vi "SACB v0.1.vi"(6 "timeout":i32=50, 7 "Command":enum16{"Create", "Read", "Close"}(ring), 8 "Error In":errorcluster, 11 "Model Name":T1) -> (0 "Error Out":errorcluster, 2 "Connected?":bool, 3 "Digital Inputs":T2)   [LabVIEW 2017]
uses:
  <vilib>/Modbus/master/Modbus Master.lvclass
  <vilib>/Modbus/master/Create Master Instance (TCP).vi
  controls/Model Name.ctl
  controls/SACB DI.ctl
panel:
  out "register values":u16[][](array[numeric])
  # "RS_Clamping_top_Front\nRS_Clamping_bottom_Front\nRS_Clamping_MotorLH_Front\nRS_Clamping_MotorRH_Front\nIPS_Part presence_top_LH\nIPS_Part presence_Bottom_LH\nIPS_Part presence_top_RH\nIPS_Part presence_Bottom_RH\nIPS_Load engaged_1\nIPS_Part presence_2\nIPS_Load engaged_MCO_LH\nIPS_Load engaged_MCO_RH"
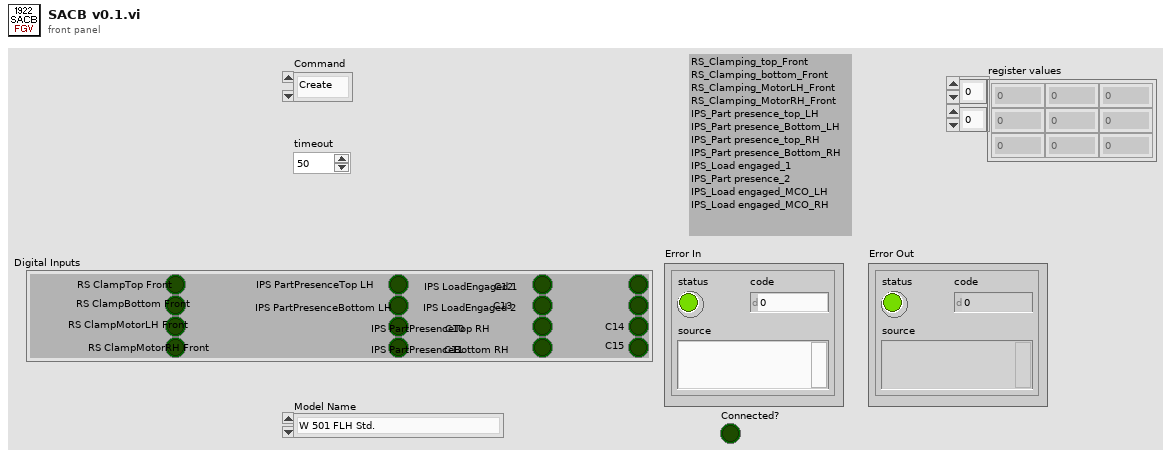
[diagram p1: front panel]
types:
  T1 = typedef "Model Name.ctl" = enum16{"W 501 FLH Std.", "W 501 FRH Std.", "W 601 FR RH Std", "W 601 FR LH Std", "W 601 RR RH Std", "W 601 RR LH Std", "W 601 FR RH AP", "W 601 FR LH AP", "W 601 RR RH AP", "W 601 RR LH AP"}
  T2 = typedef "SACB DI.ctl" = cluster{"RS ClampTop Front":bool, "RS ClampBottom Front":bool, "RS ClampMotorLH Front":bool, "RS ClampMotorRH Front":bool, "IPS PartPresenceTop LH":bool, "IPS PartPresenceBottom LH":bool, "IPS PartPresenceTop RH":bool, "IPS PartPresenceBottom RH":bool, "IPS LoadEngaged 1":bool, "IPS LoadEngaged 2":bool, "C10":bool, "C11":bool, "C12":bool, "C13":bool, "C14":bool, "C15":bool}
  T3 = cluster{"[0]":bool, "[1]":bool, "[2]":bool, "[3]":bool, "[4]":bool, "[5]":bool, "[6]":bool, "[7]":bool, "[8]":bool, "[9]":bool, "[10]":bool, "[11]":bool, "[12]":bool, "[13]":bool, "[14]":bool, "[15]":bool}
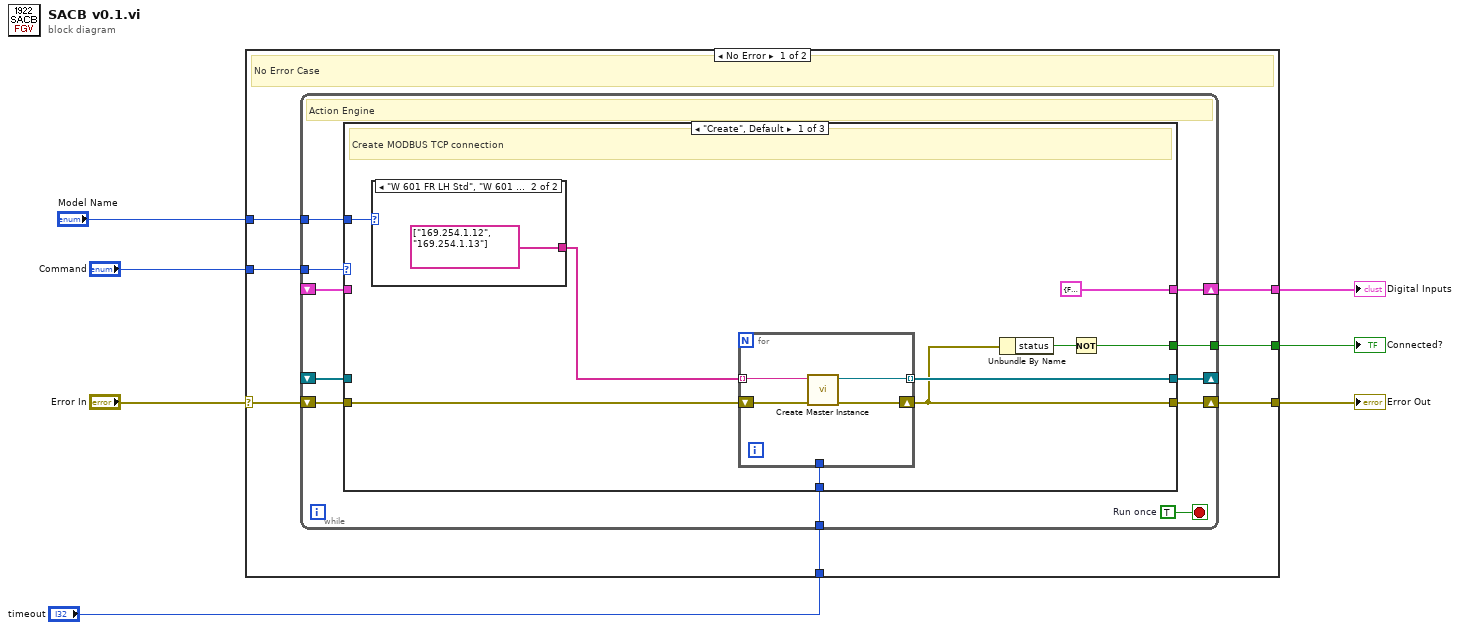
[diagram p0: block diagram]
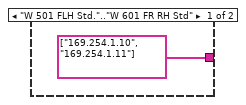
[diagram p2: hidden frame]
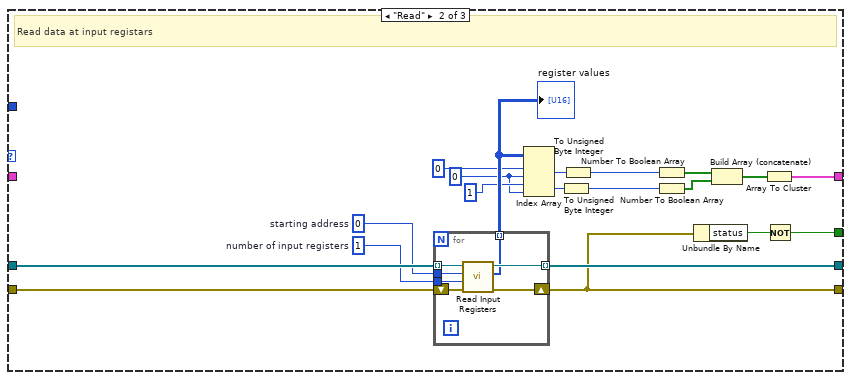
[diagram p3: hidden frame]
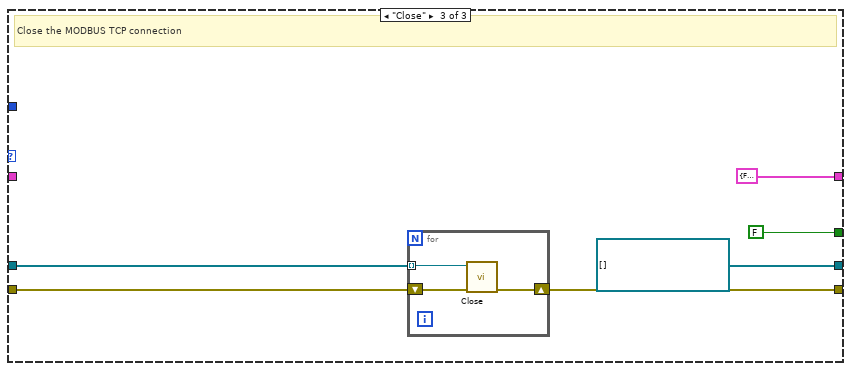
[diagram p4: hidden frame]
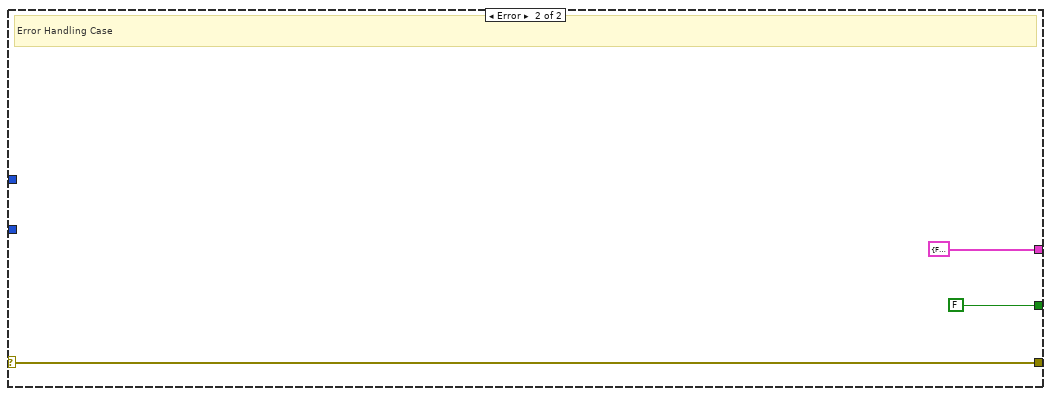
[diagram p5: hidden frame]
diagram:
  n1 = case shown="No Error" "Error In" {
    selector: "Error In" -> [w13 w79]
    tunnel: [w14 w79] -> w6
    tunnel: "Command" -> [w12 _]
    tunnel: [w11 T3 {"[0]"=FALSE, "[1]"=FALSE, "[2]"=FALSE, "[3]"=FALSE, "[4]"=FALSE, "[5]"=FALSE, "[6]"=FALSE, "[7]"=FALSE, "[8]"=FALSE, "[9]"=FALSE, "[10]"=FALSE, "[11]"=FALSE, "[12]"=FALSE, "[13]"=FALSE, "[14]"=FALSE, "[15]"=FALSE}] -> w4
    tunnel: [w10 FALSE] -> w3
    tunnel: "timeout" -> [w9 _]
    tunnel: "Model Name" -> [w8 _]
    frame No Error {
      # "No Error Case"
      n2 = while {
        tunnel: w12 -> [w23]
        shift-right: [w25] -> w14
        shift-left: w13 -> [w24]
        shift-right: [w21] -> _
        shift-left: _ -> [w20]
        shift-right: [w19] -> w11
        shift-left: _ -> [w18]
        tunnel: [w17] -> w10
        tunnel: w9 -> [w16]
        tunnel: w8 -> [w15]
        stop <- w22 stop-if-true
        w22 = TRUE  # Run once
        # "Action Engine"
        n3 = case shown="\"Create\", Default" w23 {
          tunnel: [w31 w46 w72] -> w25
          tunnel: w24 -> [w34 w60 w73]
          tunnel: [w33 w59 refnum<class "Modbus Master.lvclass">[] []] -> w21
          tunnel: w20 -> [_ w58 w71]
          tunnel: [T3 {"[0]"=FALSE, "[1]"=FALSE, "[2]"=FALSE, "[3]"=FALSE, "[4]"=FALSE, "[5]"=FALSE, "[6]"=FALSE, "[7]"=FALSE, "[8]"=FALSE, "[9]"=FALSE, "[10]"=FALSE, "[11]"=FALSE, "[12]"=FALSE, "[13]"=FALSE, "[14]"=FALSE, "[15]"=FALSE} w48 T3 {"[0]"=FALSE, "[1]"=FALSE, "[2]"=FALSE, "[3]"=FALSE, "[4]"=FALSE, "[5]"=FALSE, "[6]"=FALSE, "[7]"=FALSE, "[8]"=FALSE, "[9]"=FALSE, "[10]"=FALSE, "[11]"=FALSE, "[12]"=FALSE, "[13]"=FALSE, "[14]"=FALSE, "[15]"=FALSE}] -> w19
          tunnel: w18 -> [_ _ _]
          tunnel: [w29 w45 FALSE] -> w17
          tunnel: w16 -> [w28 _ _]
          tunnel: w15 -> [w26 _ _]
          frame "Create", Default {
            # "Create MODBUS TCP connection"
            n4 = case shown="\"W 601 FR LH Std\", \"W 601 RR RH Std\"" w26 {
              tunnel: [string[] ["169.254.1.10", "169.254.1.11"] string[] ["169.254.1.12", "169.254.1.13"]] -> w27
              frame "W 501 FLH Std.".."W 601 FR RH Std" {
              }
              frame "W 601 FR LH Std", "W 601 RR RH Std" {
              }
            }
            n5 = for {
              tunnel: [w36] -> w33 mode=indexing
              shift-right: [w38] -> w31
              shift-left: w34 -> [w37]
              tunnel: w27 -> [w35] mode=indexing
              tunnel: w28 -> [_]
              n6 = call-poly <vilib>:"Create Master Instance.vi"("error in (no error)"=w37, "address"=w35) -> ("error out"=w38:errorcluster, "TCP master instance"=w36:refnum<class "Modbus Master.lvclass">)  [unwired: 8 in]
            }
            n7 = Unbundle By Name(w31) -> ("status"=w30:bool)
            n8 = Not(x=w30) -> (.not. x?=w29:bool)
          }
          frame "Read" {
            w43 = 0 ("disabled index (col)")
            w56 = u16 1  # number of input registers
            w57 = u16 0  # starting address
            # "Read data at input registars"
            n9 = for {
              tunnel: [w65] -> w59 mode=indexing
              tunnel: w58 -> [w64] mode=indexing
              tunnel: w57 -> [w63]
              tunnel: w56 -> [w62]
              tunnel: [w61] -> w53 mode=indexing
              shift-right: [w66] -> w46
              shift-left: w60 -> [w67]
              n10 = call-dynamic "Read Input Registers.vi"("error in (no error)"=w67, "number of input registers"=w62, "starting address"=w63, "Modbus master in"=w64) -> ("error out"=w66:errorcluster, "register values"=w61:u16[], "Modbus master out"=w65:refnum<class "Modbus Master.lvclass">)  [unwired: 5 in]
            }
            "register values" <- w53
            n11 = Index Array(array=w53, index (row) #1=0 ("index"), index (col) #1=w43, index (row) #2=1 ("disabled index (col)"), index (col) #2=w43) -> (element #1=w54:u16, element #2=w51:u16)
            n12 = To Unsigned Byte Integer(number=w51) -> (unsigned 8bit integer=w41:u8)
            n13 = To Unsigned Byte Integer(number=w54) -> (unsigned 8bit integer=w42:u8)
            n14 = Number To Boolean Array(number=w42) -> (Boolean array=w55:bool[])
            n15 = Number To Boolean Array(number=w41) -> (Boolean array=w49:bool[])
            n16 = Unbundle By Name(w46) -> ("status"=w47:bool)
            n17 = Build Array (concatenate)(w55, w49) -> (w50:bool[])
            n18 = Array To Cluster(array=w50) -> (cluster=w48:T3)
            n19 = Not(x=w47) -> (.not. x?=w45:bool)
          }
          frame "Close" {
            # "Close the MODBUS TCP connection"
            n20 = for {
              tunnel: w71 -> [w74] mode=indexing
              shift-right: [w75] -> w72
              shift-left: w73 -> [w76]
              n21 = call-dynamic "Close.vi"("error in (no error)"=w76, "Modbus master in"=w74) -> ("error out"=w75:errorcluster)  [unwired: 9 in]
            }
          }
        }
      }
    }
    frame Error {
      # "Error Handling Case"
    }
  }
  "Error Out" <- w6
  "Digital Inputs" <- w4
  "Connected?" <- w3
